vi "pressure_ut_test_gauge.vi"(8 "Error In":errorcluster, 11 "Manometr in":T2) -> (0 "Error Out":errorcluster, 3 "Manometr out":T2)   [LabVIEW 2018]
uses:
  PressureGaugeInfo.ctl
  <vilib>/Utility/miscctls.llb/LVDateTimeRec.ctl
  MOKO_LabViewLibrary/MokoSTM/MokoClassicUtilitySTM/MCUS_STM.ctl
  MOKO_LabViewLibrary/MokoSTM/MokoClassicUtilitySTM/MCUS_ITEM.ctl
panel:
  in  "Минимальное значение":i64 caption="Минимальное значение на шкале прибора:"
  in  "Наименование СИ:":string
  in  "Производственный № прибора:":string
  in  "Пределы допускаемой погрешости D=±:":dbl min=0.0 format="%#_4f"
  in  "№ прибора:":dbl
  out "date time rec":T1
  in  "Драйвер:":string(combo)="0,4"
  in  "№ протокола":string caption="№ протокола:"
  in  "ММ":string(combo)
  in  "ДД":i64=1 min=1 max=31
  in  "ГГГГ":dbl=1.0 caption="ГГГГ:"
  in  "Давление":dbl caption="Давление окружающей среды, мм. рт. ст.:"
  in  "Цена деления":dbl caption="Цена деления:" format="%#_4g"
  in  "Температура":dbl caption="Температура окружающего воздуха, °С:"
  in  "Влажность":dbl caption="Относительная влажность воздуха, %:"
  in  "Номер заказа":string caption="Номер заказа:"
  in  "Номер рабочего места":string caption="Номер рабочего места:"
  in  "ФИО":string caption="Поверку провел:"
  in  "Место проведения":string caption="Место проведения поверки:"
  in  "Владелец":string caption="Владелец:"
  in  "Номер клейма":string caption="Номер клейма:"
  in  "Тип":string caption="Тип:"
  in  "Первая точка":dbl=1.0 caption="Первая поверяемая точка на шкале прибора после нуля:" format="%#_3f"
  in  "Предельное давление":dbl=1.0 caption="Предельное значение давления на шкале прибора:" format="%#_3f"
  in  "Класс точности:":string(combo)="0,4"
  in  "Единица измерения:":string(combo)="kPa"
  in  "Применить":bool
  # "!\"№;%:?*()_+ЙЦУКЕНГ?*Ш(ЩЗХЪ\nФЫВАПРОЛДЖЭ\nЯЧСМИТЬБЮ,"
  # "Информация об образце"
  # "Информация о поверке"
  # "0,4\n0,6\n1\n1,5\n1,6\n2,5\n4"
  # "kPa\nbar\nkgf/cm2\nMPa"
  # "Характеристики манометра"
  # "Условия поверки"
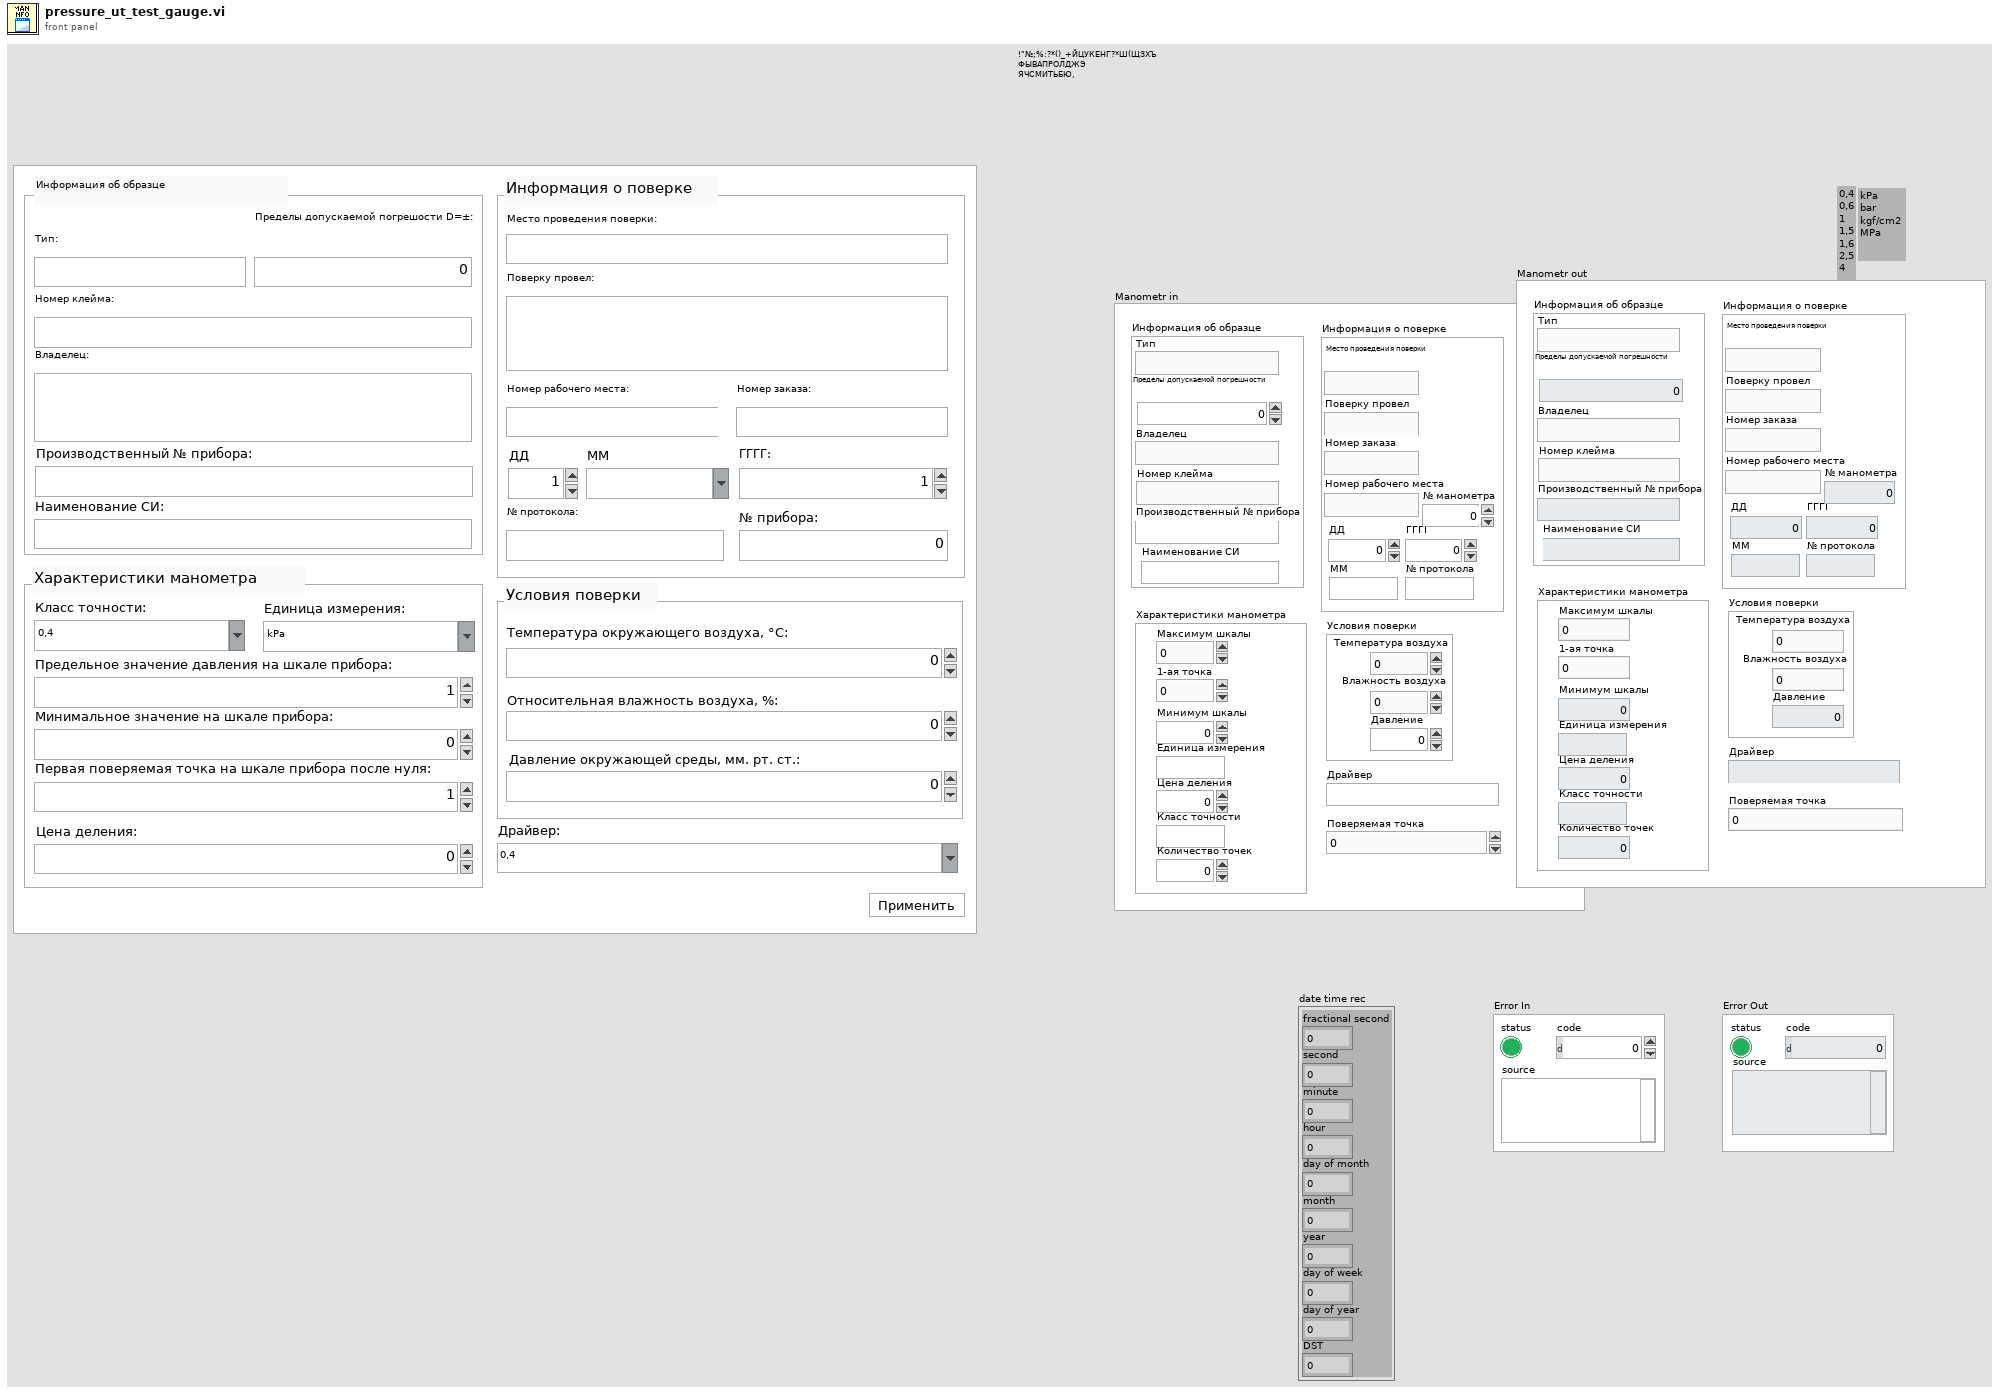
[diagram p1: front panel]
types:
  T1 = typedef "LVDateTimeRec.ctl" = cluster{"fractional second":dbl, "second":i32, "minute":i32, "hour":i32, "day of month":i32, "month":i32, "year":i32, "day of week":i32, "day of year":i32, "DST":i32}
  T2 = typedef "PressureGaugeInfo.ctl" = cluster{"Информация об образце":cluster{"Тип":string, "Владелец":string, "Номер клейма":string, "Пределы допускаемой погрешности ":dbl, "Производственный № прибора":string, "Наименование СИ":string}, "Информация о поверке":cluster{"Место проведения поверки":string, "Поверку провел":string, "Номер заказа":string, "Номер рабочего места":string, "ДД":dbl, "ММ":string, "ГГГГ":dbl, "№ протокола":string, "№ манометра":dbl}, "Характеристики манометра":cluster{"Максимум шкалы":dbl, "1-ая точка":dbl, "Единица измерения":string, "Цена деления":dbl, "Класс точности":string, "Минимум шкалы":dbl, "Количество точек":dbl}, "Условия поверки":cluster{"Температура воздуха":dbl, "Влажность воздуха":dbl, "Давление":dbl}, "Драйвер":string, "Поверяемая точка":dbl}
  T3 = typedef "MCUS_STM.ctl" = cluster{"main stm":T4, "data":string}
  T4 = typedef "MCUS_ITEM.ctl" = enum16{"idle", "_____ main_____ ", "Init", "Stop", "Apply values"}
  T5 = cluster{"Максимум шкалы":dbl, "1-ая точка":dbl, "Единица измерения":string, "Цена деления":dbl, "Класс точности":string, "Минимум шкалы":dbl, "Количество точек":dbl}
  T6 = cluster{"Температура воздуха":dbl, "Влажность воздуха":dbl, "Давление":dbl}
  T7 = cluster{"Тип":string, "Владелец":string, "Номер клейма":string, "Пределы допускаемой погрешности ":dbl, "Производственный № прибора":string, "Наименование СИ":string}
  T8 = cluster{"Место проведения поверки":string, "Поверку провел":string, "Номер заказа":string, "Номер рабочего места":string, "ДД":dbl, "ММ":string, "ГГГГ":dbl, "№ протокола":string, "№ манометра":dbl}
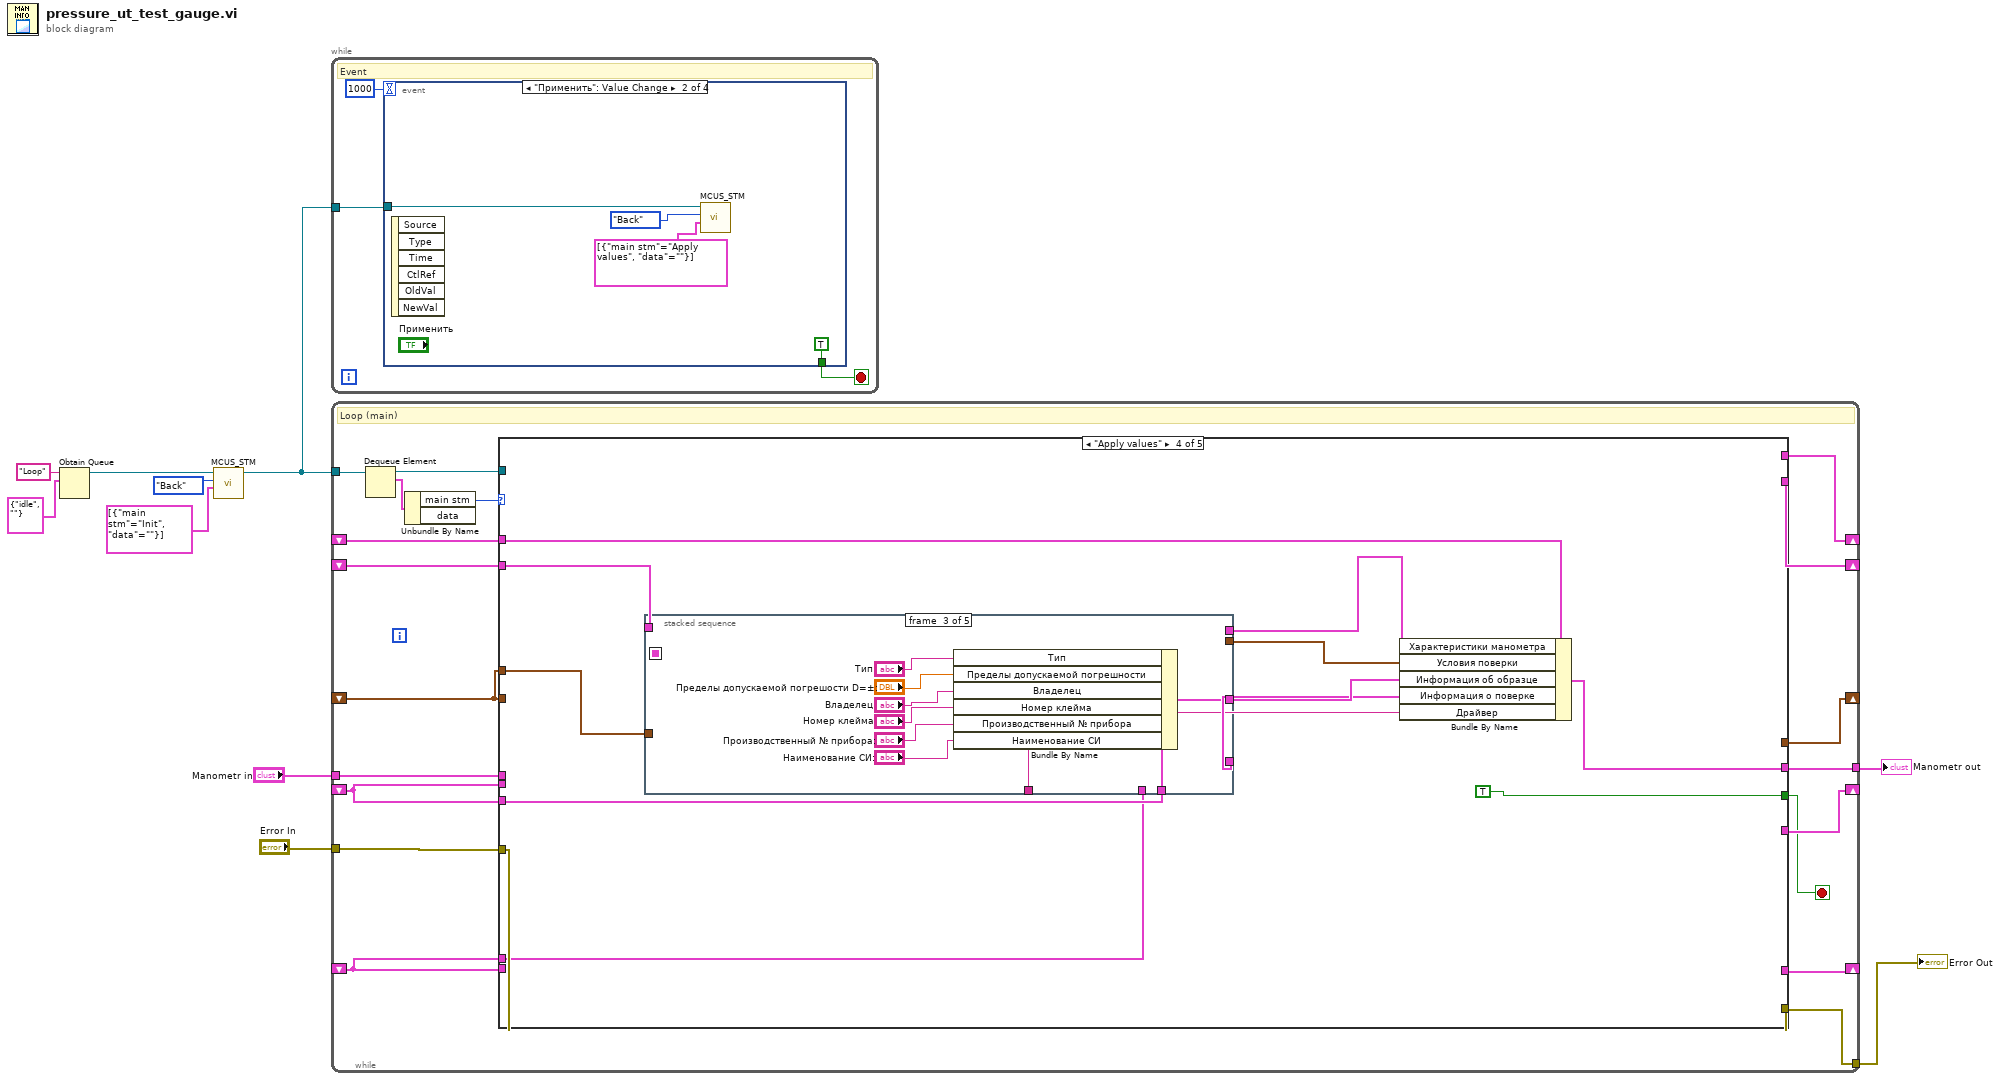
[diagram p0: block diagram]
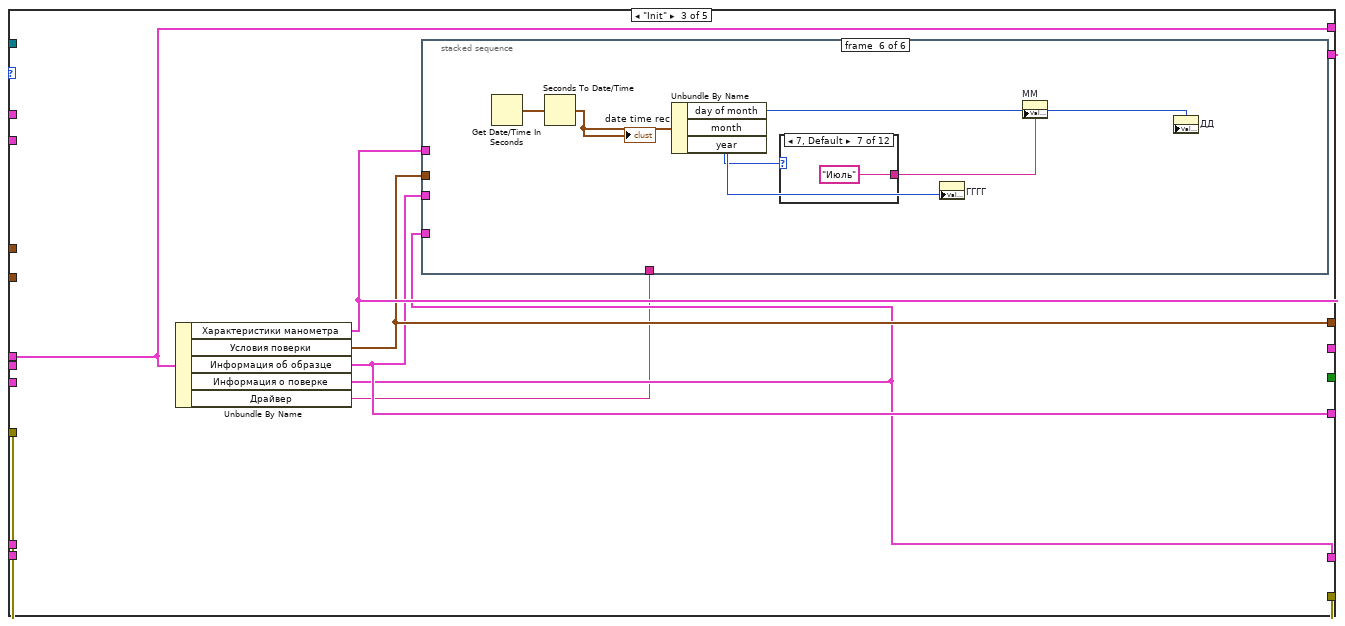
[diagram p4: hidden frame]
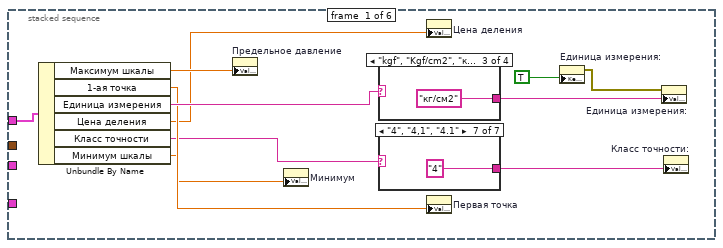
[diagram p5: hidden frame]
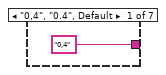
[diagram p6: hidden frame]
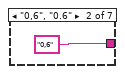
[diagram p7: hidden frame]
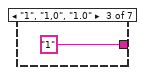
[diagram p8: hidden frame]
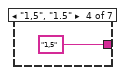
[diagram p9: hidden frame]
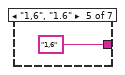
[diagram p10: hidden frame]
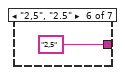
[diagram p11: hidden frame]
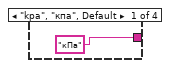
[diagram p12: hidden frame]
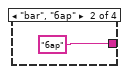
[diagram p13: hidden frame]
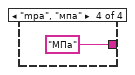
[diagram p14: hidden frame]
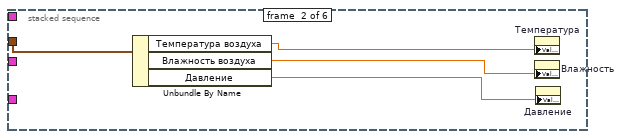
[diagram p15: hidden frame]
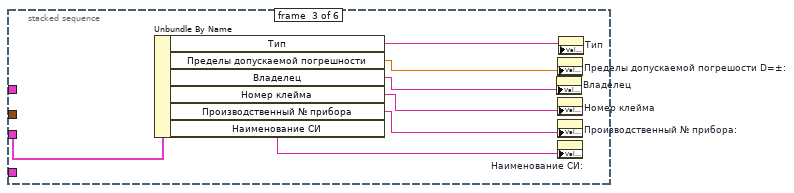
[diagram p16: hidden frame]
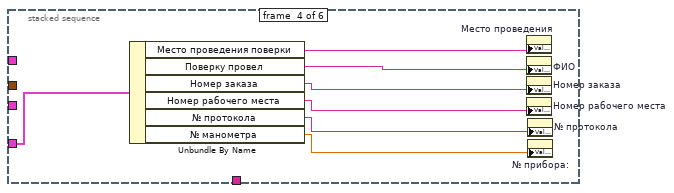
[diagram p17: hidden frame]
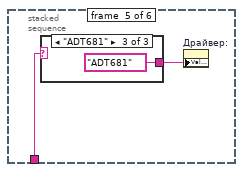
[diagram p18: hidden frame]
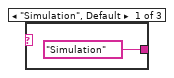
[diagram p19: hidden frame]
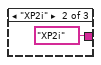
[diagram p20: hidden frame]
diagram:
  n1 = Obtain Queue(name (unnamed)="Loop", element data type=T3 {"main stm"=enum."idle", "data"=""} ("MOKO_NMEA")) -> (queue out=w10:refnum<queue>)  [unwired: 3 in, 2 out]
  n2 = call "MCUS_STM.vi"("StateMachineSteps"=T3[] [{"main stm"=enum."Init", "data"=""}], "FNs"=enum16{"Back", "Front", "Replace"}."Back", "Queue in"=w10) -> ("Queue out"=w5:refnum<queue>)  [unwired: 7 in, 1 out]
  n3 = while {
    tunnel: w5 -> [w11]
    stop <- w13 stop-if-true
    # "Event"
    n4 = event shown="[1] \"Применить\": Value Change" {
      selector: _ -> [_ _ _ _]
      dyn-events: _ -> [_ _ _ _]
      timeout: 1000 -> [_ _ _ _]
      tunnel: [_ TRUE _ TRUE] -> w13
      tunnel: w11 -> [_ w16 _ w18]
      event Timeout {
        n5 = event-data() -> ()  [unwired: 1 in, 3 out]
      }
      event "Применить": Value Change {
        n6 = event-data() -> ()  [unwired: 1 in, 6 out]
        n7 = call "MCUS_STM.vi"("StateMachineSteps"=T3[] [{"main stm"=enum."Apply values", "data"=""}], "FNs"=enum16{"Back", "Front", "Replace"}."Back", "Queue in"=w16) -> ()  [unwired: 7 in, 2 out]
      }
      event "Единица измерения:", "Класс точности:", "Предельное давление", "Первая точка", "Тип", "Номер клейма", "Владелец", "Место проведения", "ФИО", "Номер рабочего места", "Номер заказа", "Влажность", "Температура", "Цена деления", "Давление", "ГГГГ", "ДД", "ММ": Value Change {
        n8 = event-data() -> ()  [unwired: 1 in, 6 out]
      }
      event Panel Close {
        n9 = event-data() -> ()  [unwired: 1 in, 4 out]
        n10 = call "MCUS_STM.vi"("StateMachineSteps"=T3[] [{"main stm"=enum."Stop", "data"=""}], "FNs"=enum16{"Back", "Front", "Replace"}."Replace", "Queue in"=w18) -> ()  [unwired: 7 in, 2 out]
      }
    }
  }
  n11 = while {
    tunnel: w5 -> [w40]
    shift-right: [w36] -> _
    shift-left: _ -> [w35]
    shift-right: [w34] -> _
    shift-left: _ -> [w24]
    shift-right: [w33] -> _
    shift-left: _ -> [w23]
    shift-right: [w32] -> _
    shift-left: _ -> [w22]
    shift-right: [w31] -> _
    shift-left: _ -> [w29]
    tunnel: [w28] -> w4
    tunnel: "Manometr in" -> [w27]
    tunnel: "Error In" -> [w26]
    tunnel: [w25] -> w1
    stop <- w30 stop-if-true
    # "Loop (main)"
    n12 = Dequeue Element(queue=w40) -> (queue out=w39:refnum<queue>, element=w38:T3)  [unwired: 2 in, 2 out]
    n13 = Unbundle By Name(w38) -> ("main stm"=w37:T4)  [unwired: 1 out]
    n14 = case shown="\"Apply values\"" w37 {
      tunnel: w39 -> [_ _ _ _ _]
      tunnel: [w44 _ w50 _ w168] -> w36
      tunnel: w35 -> [w44 _ _ w124 w168]
      tunnel: [w43 _ w49 _ w167] -> w34
      tunnel: w24 -> [w43 _ _ _ w167]
      tunnel: [w42 _ w48 _ w165] -> w33
      tunnel: w23 -> [w42 _ _ _ w165]
      tunnel: [w41 _ w47 _ w164] -> w32
      tunnel: w22 -> [w41 _ _ _ w164]
      tunnel: [w45 _ w52 _ w169] -> w31
      tunnel: w29 -> [w45 _ _ w128 w169]
      tunnel: [_ _ _ TRUE TRUE] -> w30
      tunnel: [_ _ _ w126 w166] -> w28
      tunnel: w27 -> [_ _ w52 _ w166]
      tunnel: w26 -> [_ _ w51 w125 w163]
      tunnel: [_ _ w51 w125 w163] -> w25
      tunnel: w24 -> [_ _ _ w122 _]
      tunnel: w23 -> [_ _ _ w120 _]
      tunnel: w22 -> [_ _ _ w118 _]
      frame "idle", Default {
      }
      frame "_____ main_____ " {
      }
      frame "Init" {
        n15 = Unbundle By Name(w52) -> ("Характеристики манометра"=w50:T5, "Условия поверки"=w49:T6, "Информация об образце"=w48:T7, "Информация о поверке"=w47:T8, "Драйвер"=w46:string)
        n16 = stacked-sequence {
          tunnel: w50 -> [w59 _ _ _ _ _]
          tunnel: w49 -> [_ w75 _ _ _ _]
          tunnel: w48 -> [_ _ w79 _ _ _]
          tunnel: w47 -> [_ _ _ w86 _ _]
          tunnel: w46 -> [_ _ _ _ w93 _]
          frame #0 {
            n17 = Unbundle By Name(w59) -> ("Максимум шкалы"=w58:dbl, "1-ая точка"=w56:dbl, "Единица измерения"=w57:string, "Цена деления"=w55:dbl, "Класс точности"=w54:string, "Минимум шкалы"=w53:dbl)
            n18 = property on="Предельное давление" class="DigNum (strict)"("Value"=w58) -> ()  [unwired: 2 in, 2 out]
            n19 = property on="Минимум" class="DigNum (strict)"("Val(Sgnl)"=w53) -> ()  [unwired: 2 in, 2 out]
            n20 = case shown="\"kgf\", \"Kgf/cm2\", \"кг/см2\"" w57 {
              tunnel: ["кПа" "бар" "кг/см2" "МПа"] -> w63
              frame "kpa", "кпа", Default {
              }
              frame "bar", "бар" {
              }
              frame "kgf", "Kgf/cm2", "кг/см2" {
              }
              frame "mpa", "мпа" {
              }
            }
            n21 = case shown="\"4\", \"4,1\", \"4.1\"" w54 {
              tunnel: ["0,4" "0,6" "1" "1,5" "1,6" "2,5" "4"] -> w60
              frame "0,4", "0.4", Default {
              }
              frame "0,6", "0.6" {
              }
              frame "1", "1,0", "1.0" {
              }
              frame "1,5", "1.5" {
              }
              frame "1,6", "1.6" {
              }
              frame "2,5", "2.5" {
              }
              frame "4", "4,1", "4.1" {
              }
            }
            n22 = property on="Цена деления" class="DigNum (strict)"("Value"=w55) -> ()  [unwired: 2 in, 2 out]
            n23 = property on="Первая точка" class="DigNum (strict)"("Value"=w56) -> ()  [unwired: 2 in, 2 out]
            n24 = property on="Единица измерения:" class="CmbBox"("Key Focus"=TRUE) -> (error out=w61:errorcluster)  [unwired: 2 in, 1 out]
            n25 = property on="Единица измерения:" class="CmbBox"(error in=w61, "Value"=w63) -> ()  [unwired: 1 in, 2 out]
            n26 = property on="Класс точности:" class="CmbBox"("Value"=w60) -> ()  [unwired: 2 in, 2 out]
          }
          frame #1 {
            n27 = Unbundle By Name(w75) -> ("Температура воздуха"=w76:dbl, "Влажность воздуха"=w77:dbl, "Давление"=w78:dbl)
            n28 = property on="Температура" class="DigNum (strict)"("Value"=w76) -> ()  [unwired: 2 in, 2 out]
            n29 = property on="Влажность" class="DigNum (strict)"("Value"=w77) -> ()  [unwired: 2 in, 2 out]
            n30 = property on="Давление" class="DigNum (strict)"("Value"=w78) -> ()  [unwired: 2 in, 2 out]
          }
          frame #2 {
            n31 = Unbundle By Name(w79) -> ("Тип"=w80:string, "Пределы допускаемой погрешности"=w83:dbl, "Владелец"=w81:string, "Номер клейма"=w82:string, "Производственный № прибора"=w84:string, "Наименование СИ"=w85:string)
            n32 = property on="Владелец" class="Str"("Value"=w81) -> ()  [unwired: 2 in, 2 out]
            n33 = property on="Пределы допускаемой погрешости D=±:" class="DigNum (strict)"("Val(Sgnl)"=w83) -> ()  [unwired: 2 in, 2 out]
            n34 = property on="Номер клейма" class="Str"("Value"=w82) -> ()  [unwired: 2 in, 2 out]
            n35 = property on="Производственный № прибора:" class="Str"("Value"=w84) -> ()  [unwired: 2 in, 2 out]
            n36 = property on="Наименование СИ:" class="Str"("Value"=w85) -> ()  [unwired: 2 in, 2 out]
            n37 = property on="Тип" class="Str"("Value"=w80) -> ()  [unwired: 2 in, 2 out]
          }
          frame #3 {
            n38 = Unbundle By Name(w86) -> ("Место проведения поверки"=w87:string, "Поверку провел"=w88:string, "Номер заказа"=w89:string, "Номер рабочего места"=w90:string, "№ протокола"=w91:string, "№ манометра"=w92:dbl)
            n39 = property on="Место проведения" class="Str"("Value"=w87) -> ()  [unwired: 2 in, 2 out]
            n40 = property on="ФИО" class="Str"("Value"=w88) -> ()  [unwired: 2 in, 2 out]
            n41 = property on="Номер заказа" class="Str"("Value"=w89) -> ()  [unwired: 2 in, 2 out]
            n42 = property on="Номер рабочего места" class="Str"("Value"=w90) -> ()  [unwired: 2 in, 2 out]
            n43 = property on="№ протокола" class="Str"("Value"=w91) -> ()  [unwired: 2 in, 2 out]
            n44 = property on="№ прибора:" class="DigNum (strict)"("Value"=w92) -> ()  [unwired: 2 in, 2 out]
          }
          frame #4 {
            n45 = case shown="\"ADT681\"" w93 {
              tunnel: ["Simulation" ("Драйвер:") "XP2i" ("Драйвер:") "ADT681" ("Драйвер:")] -> w94
              frame "Simulation", Default {
              }
              frame "XP2i" {
              }
              frame "ADT681" {
              }
            }
            n46 = property on="Драйвер:" class="CmbBox"("Value"=w94) -> ()  [unwired: 2 in, 2 out]
          }
          frame #5 {
            n47 = Get Date/Time In Seconds() -> (seconds since 1Jan1904=w98:timestamp)
            n48 = Seconds To Date/Time(time stamp (now)=w98) -> (date time rec=w99:T1)  [unwired: 1 in]
            "date time rec" <- w99
            n49 = Unbundle By Name(w99) -> ("day of month"=w100:i32, "month"=w101:i32, "year"=w103:i32)
            n50 = case shown="7, Default" w101 {
              tunnel: ["Январь" "Февраль" "Март" "Апрель" "Май" "Июнь" "Июль" "Август" "Сентябрь" "Октябрь" "Ноябрь" "Декабрь"] -> w102
              frame 1 {
              }
              frame 2 {
              }
              frame 3 {
              }
              frame 4 {
              }
              frame 5 {
              }
              frame 6 {
              }
              frame 7, Default {
              }
              frame 8 {
              }
              frame 9 {
              }
              frame 10 {
              }
              frame 11 {
              }
              frame 12 {
              }
            }
            n51 = property on="ГГГГ" class="DigNum (strict)"("Value"=w103) -> ()  [unwired: 2 in, 2 out]
            n52 = property on="ММ" class="CmbBox"("Value"=w102) -> ()  [unwired: 2 in, 2 out]
            n53 = property on="ДД" class="DigNum (strict)"("Value"=w100) -> ()  [unwired: 2 in, 2 out]
          }
        }
      }
      frame "Apply values" {
        n54 = stacked-sequence {
          seq-local: [w135 _ _ _ _] -> [_ w142 _ _ _]
          tunnel: w124 -> [w136 _ _ _ _]
          tunnel: [_ w142 _ _ _] -> w123
          tunnel: w122 -> [_ w138 _ _ _]
          tunnel: [_ w137 _ _ _] -> w121
          tunnel: w120 -> [_ _ w144 _ _]
          tunnel: [_ _ w143 _ _] -> w119
          tunnel: w118 -> [_ _ _ w152 _]
          tunnel: [_ _ _ w151 _] -> w117
          tunnel: [_ _ _ _ "Драйвер:"] -> w116
          frame #0 {
            n55 = Bundle By Name(cluster=w136, "Максимум шкалы"="Предельное давление", "1-ая точка"="Первая точка", "Единица измерения"="Единица измерения:", "Цена деления"="Цена деления", "Класс точности"="Класс точности:", "Минимум шкалы"="Минимальное значение") -> (w135:T5)
          }
          frame #1 {
            n56 = Bundle By Name(cluster=w138, "Температура воздуха"="Температура", "Влажность воздуха"="Влажность", "Давление"="Давление") -> (w137:T6)
          }
          frame #2 {
            n57 = Bundle By Name(cluster=w144, "Тип"="Тип", "Пределы допускаемой погрешности"="Пределы допускаемой погрешости D=±:", "Владелец"="Владелец", "Номер клейма"="Номер клейма", "Производственный № прибора"="Производственный № прибора:", "Наименование СИ"="Наименование СИ:") -> (w143:T7)
          }
          frame #3 {
            n58 = Bundle By Name(cluster=w152, "Место проведения поверки"="Место проведения", "Поверку провел"="ФИО", "Номер заказа"="Номер заказа", "Номер рабочего места"="Номер рабочего места", "ДД"="ДД", "ММ"="ММ", "ГГГГ"="ГГГГ", "№ протокола"="№ протокола", "№ манометра"="№ прибора:") -> (w151:T8)
          }
          frame #4 {
          }
        }
        n59 = Bundle By Name(cluster=w128, "Характеристики манометра"=w123, "Условия поверки"=w121, "Информация об образце"=w119, "Информация о поверке"=w117, "Драйвер"=w116) -> (w126:T2)
      }
      frame "Stop" {
      }
    }
  }
  "Manometr out" <- w4
  "Error Out" <- w1
